vi "REQ Initialize Hardware.vi"(6 "wait for reply (T)":bool=TRUE, 8 "error in":errorcluster, 9 "Connection Ref":variant, 10 "Session Setting":T1={"cluster (:memory:)"=":memory:", "interface"=""}) -> (0 "error out":errorcluster, 1 "timed out?":bool, 3 "Connect?":bool)   [LabVIEW 2021, in "CAN.lvlib"]
doc: "_____\nCreated using DQMH Event Scripter 6.1.0.128."
uses:
  CAN.lvlib
  REQ Initialize Hardware Argument--cluster.ctl
  REQ Initialize Hardware (Reply Payload)--cluster.ctl
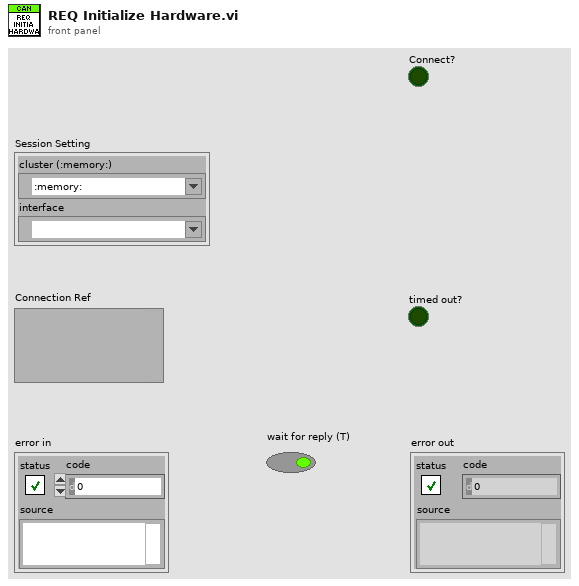
[diagram p1: front panel]
types:
  T1 = cluster{"cluster (:memory:)":refnum<k21>, "interface":refnum<k21>}
  T2 = typedef "CAN.lvlib/REQ Initialize Hardware Argument--cluster.ctl" = cluster{"Session Setting":cluster{"cluster (:memory:)":refnum<k21>, "interface":refnum<k21>}, "Connection Ref":variant, "Wait Notifier":refnum<notifier>, "wait for reply":bool}
  T3 = typedef "CAN.lvlib/Request Events--cluster.ctl" = cluster{"Stop Module":refnum<user-event>, "Show Panel":refnum<user-event>, "Hide Panel":refnum<user-event>, "Get Module Execution Status":refnum<user-event>, "Show Diagram":refnum<user-event>, "REQ Initialize Hardware":refnum<user-event>, "REQ Setup":refnum<user-event>, "REQ Get Channel Data":refnum<user-event>, "REQ CAN Data":refnum<user-event>, "REQ Close Ref":refnum<user-event>, "REQ Create CAN Database":refnum<user-event>}
  T4 = typedef "CAN.lvlib/REQ Initialize Hardware (Reply Payload)--cluster.ctl" = cluster{"Connect?":bool, "error":errorcluster}
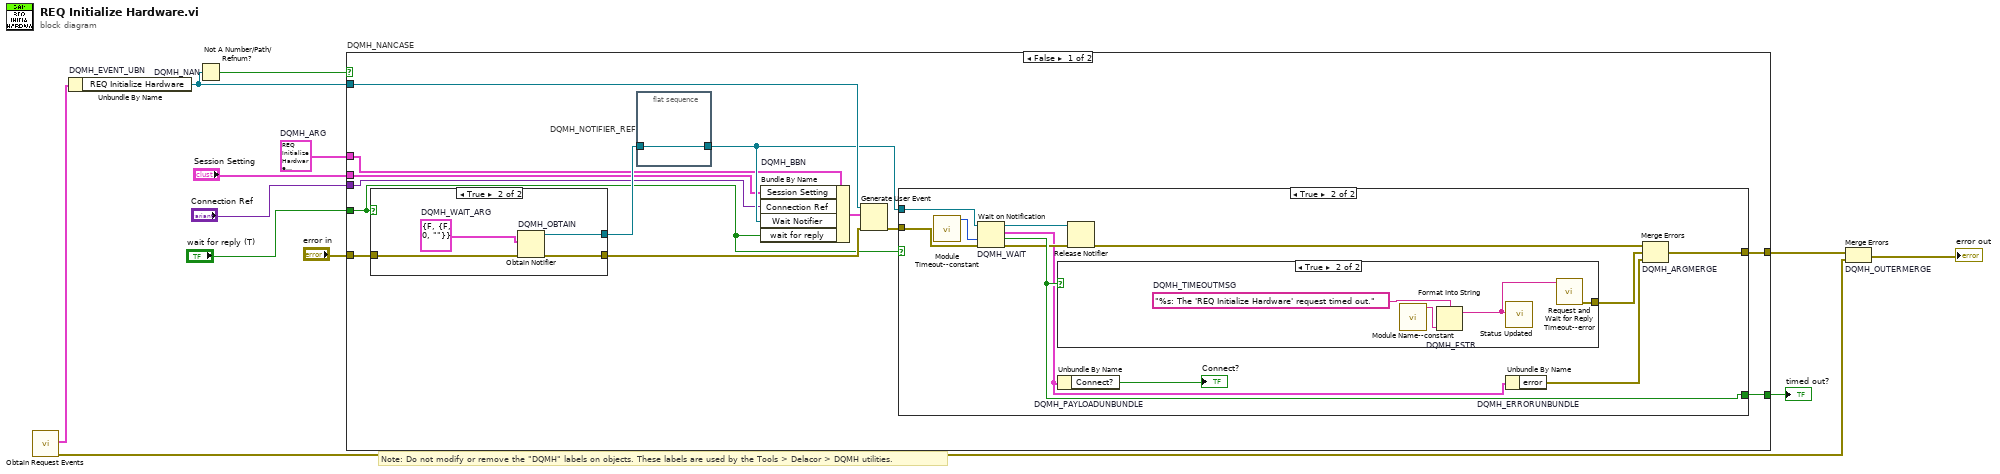
[diagram p0: block diagram]
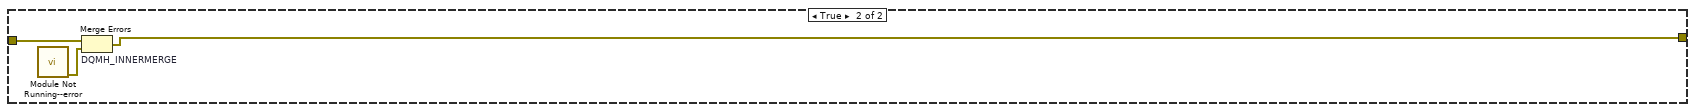
[diagram p5: hidden frame]
diagram:
  w6 = T2 {"Session Setting"={"cluster (:memory:)"=":memory:", "interface"=""}, "Connection Ref"=variant, "Wait Notifier"=refnum, "wait for reply"=FALSE}  # DQMH_ARG
  # "Note: Do not modify or remove the \"DQMH\" labels on objects. These labels are used by the Tools > Delacor > DQMH utilities."
  n1 = call "Obtain Request Events.vi"() -> ("error out"=w2:errorcluster, "CAN Request Events"=w1:T3)  [unwired: 10 in]
  n2 = Unbundle By Name "DQMH_EVENT_UBN"(w1) -> ("REQ Initialize Hardware"=w10:refnum<user-event>)
  n3 = Not A Number/Path/Refnum? "DQMH_NAN"(number/path/refnum=w10) -> (NaN/Path/Refnum?=w9:bool)
  n4 = case "DQMH_NANCASE" shown="False" w9 {
    tunnel: "error in" -> [w25 w51]
    tunnel: w10 -> [w23 _]
    tunnel: [w20 w50] -> w7
    tunnel: [w21 _] -> w8
    tunnel: w6 -> [w16 _]
    tunnel: "Session Setting" -> [w15 _]
    tunnel: "Connection Ref" -> [w14 _]
    tunnel: "wait for reply (T)" -> [w13 _]
    frame False {
      n5 = case shown="True" w13 {
        tunnel: w25 -> [w44 w48]
        tunnel: [w44 w47] -> w22
        tunnel: [_ w45] -> w18
        frame False {
        }
        frame True {
          w46 = T4 {"Connect?"=FALSE, "error"={"status"=FALSE, "code"=0, "source"=""}}  # DQMH_WAIT_ARG
          n6 = Obtain Notifier "DQMH_OBTAIN"(notification data type=w46, error in (no error)=w48) -> (notifier out=w45:refnum<notifier>, error out=w47:errorcluster)  [unwired: 2 in, 1 out]
        }
      }
      n7 = flat-sequence "DQMH_NOTIFIER_REF" {
        tunnel: w18 -> [w26]
        tunnel: [w26] -> w17
        frame #0 {
        }
      }
      n8 = Bundle By Name "DQMH_BBN"(cluster=w16, "Session Setting"=w15, "Connection Ref"=w14, "Wait Notifier"=w17, "wait for reply"=w13) -> (w19:T2)
      n9 = Generate User Event(user event=w23, event data cluster=w19, error in=w22) -> (error out=w24:errorcluster)  [unwired: 1 in, 1 out]
      n10 = case shown="True" w13 {
        tunnel: w24 -> [w27 w39]
        tunnel: w17 -> [_ w38]
        tunnel: [_ w36] -> w21
        tunnel: [w27 w35] -> w20
        frame False {
        }
        frame True {
          n11 = call "Module Timeout--constant.vi"() -> ("Module Timeout"=w29:i32)  [unwired: 11 in]
          n12 = Wait on Notification "DQMH_WAIT"(notifier=w38, timeout in ms (-1)=w29, error in (no error)=w39) -> (notifier out=w37:refnum<notifier>, notification=w30:T4, timed out?=w36:bool, error out=w34:errorcluster)  [unwired: 1 in]
          n13 = case shown="True" w36 {
            tunnel: [_ w41] -> w31
            frame False {
            }
            frame True {
              w43 = "%s: The 'REQ Initialize Hardware' request timed out."  # DQMH_TIMEOUTMSG
              n14 = call "Module Name--constant.vi"() -> ("Module Name"=w40:string)  [unwired: 11 in]
              n15 = Format Into String "DQMH_FSTR"(format string=w43, w40) -> (resulting string=w42:string)  [unwired: 2 in, 1 out]
              n16 = call "Status Updated.vi"("Status"=w42) -> ()  [unwired: 10 in, 1 out]
              n17 = call "Request and Wait for Reply Timeout--error.vi"("Error Message"=w42) -> ("error out"=w41:errorcluster)  [unwired: 10 in]
            }
          }
          n18 = Unbundle By Name "DQMH_PAYLOADUNBUNDLE"(w30) -> ("Connect?"=→"Connect?":bool)
          n19 = Release Notifier(notifier=w37, error in (no error)=w34) -> (error out=w33:errorcluster)  [unwired: 1 in, 2 out]
          n20 = Unbundle By Name "DQMH_ERRORUNBUNDLE"(w30) -> ("error"=w32:errorcluster)
          n21 = Merge Errors "DQMH_ARGMERGE"(w33, w31, w32) -> (w35:errorcluster)
        }
      }
    }
    frame True {
      n22 = call "Module Not Running--error.vi"() -> ("error out"=w49:errorcluster)  [unwired: 11 in]
      n23 = Merge Errors "DQMH_INNERMERGE"(w51, w49) -> (w50:errorcluster)
    }
  }
  "timed out?" <- w8
  n24 = Merge Errors "DQMH_OUTERMERGE"(w7, w2) -> (→"error out":errorcluster)
